vi "Open Device.vi"(8 "error in (no error)":errorcluster, 11 "ThAr in":refnum<class "ThAr.lvclass">) -> (0 "error constant":errorcluster, 2 "Handle":u32, 3 "ThAr out":refnum<class "ThAr.lvclass">)   [LabVIEW 2016, in "ThAr.lvclass"]
uses:
  ThAr.lvclass
  ThAr.lvclass/ThAr.ctl
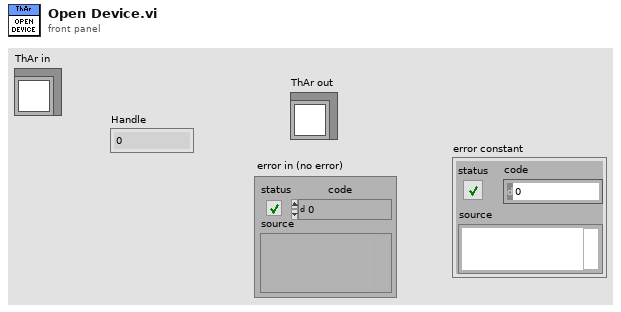
[diagram p1: front panel]
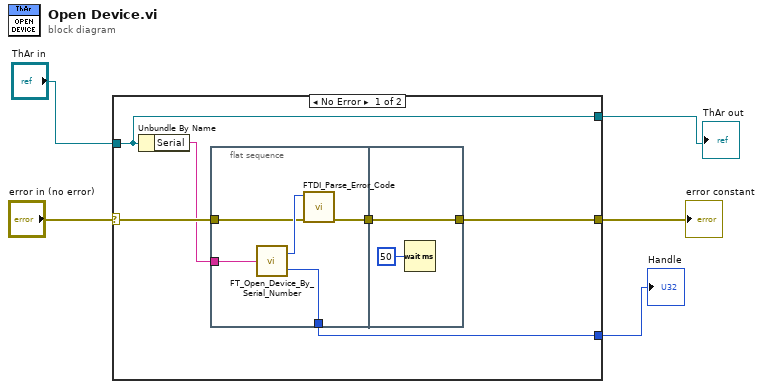
[diagram p0: block diagram]
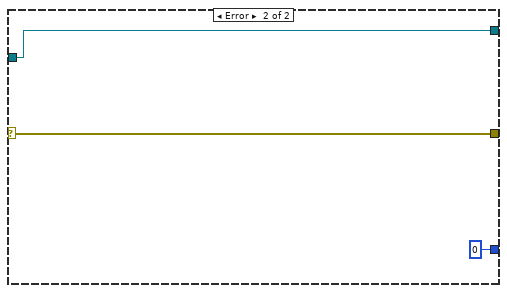
[diagram p2: hidden frame]
diagram:
  n1 = case shown="No Error" "error in (no error)" {
    selector: "error in (no error)" -> [w10 w21]
    tunnel: [w11 w21] -> w5
    tunnel: [w8 u32 0 ("Handle")] -> w3
    tunnel: "ThAr in" -> [w6 w19]
    tunnel: [w6 w19] -> w1
    frame No Error {
      n2 = Unbundle By Name(w6) -> ("Serial"=w7:string)
      n3 = flat-sequence {
        tunnel: w10 -> [w14]
        tunnel: w7 -> [w13]
        tunnel: [w15] -> w9
        tunnel: [w12] -> w8
        tunnel: [w18] -> w11
        tunnel: w9 -> [w18]
        frame #0 {
          n4 = call "FT_Open_Device_By_Serial_Number.vi"("Device Serial Number"=w13) -> ("FT_Status"=w16:u32, "Handle"=w12:u32)
          n5 = call "FTDI_Parse_Error_Code.vi"("error in (no error)"=w14, "FT_Status"=w16) -> ("error out"=w15:errorcluster)  [unwired: 9 in]
        }
        frame #1 {
          n6 = Wait (ms)(milliseconds to wait=u32 50) -> ()  [unwired: 1 out]
        }
      }
    }
    frame Error {
    }
  }
  "error constant" <- w5
  "Handle" <- w3
  "ThAr out" <- w1
